vi "Read Lockin Digitizer Configuration.vi"(8 "error in (no error)":errorcluster, 11 "DAQmx RP I-V Driver in":refnum<class "RP I-V Driver.lvclass">) -> (0 "error out":errorcluster, 2 "Configuration":T1={"Post-trigger delay"=0.01, "Post-trigger duration"=0.1, "Rate"=1000000.0, "Ranges"=[10.0], "Re-name channels"=[], "Active channels"="0:1", "External\nclock"=FALSE, "Monitor time\nconstant"=1.0, "Sync"=FALSE, "Lock-in input channel phases"=[], "Output channels configuration"=[]} {"Output channels configuration"."Output amplitude" format="%#_6pV"; "Output channels configuration"."Frequency" format="%#_6pHz"; "Monitor time\nconstant" format="%#_6ps"; "Rate" format="%#_8pHz"; "Post-trigger duration" format="%#_6ps"; "Post-trigger delay" format="%#_6ps"; "Ranges" format="%#_6pV"}, 3 "DAQmx RP I-V Driver in":refnum<class "RP I-V Driver.lvclass">)   [LabVIEW 2024, in "RP I-V Driver.lvclass"]
uses:
  RP I-V Driver.lvclass
  Instruments/Pulse Driver/Lockin Digitizer Driver/Lockin Digitizer Configuration.ctl
  RP I-V Driver.lvclass/RP I-V Driver.ctl
  Instruments/Lockin Digitizer Driver/Output Channel Configuration.ctl
panel:
  # "Pulse config"
  # "Lock-in config"
  # "Output        Output          Input\nfrequency    amplitude    channels"
  # "#0\n\n#1\n\n#3"
  # "Monitor config"
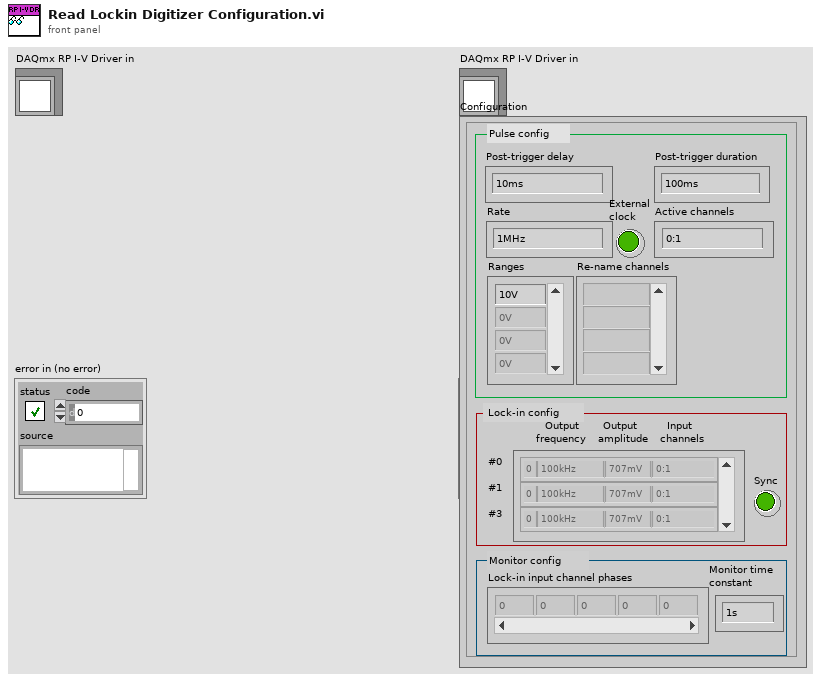
[diagram p1: front panel]
types:
  T1 = typedef "Lockin Digitizer Configuration.ctl" = cluster{"Post-trigger delay":dbl, "Post-trigger duration":dbl, "Rate":dbl, "Ranges":dbl[], "Re-name channels":string[], "Active channels":string, "External\nclock":bool, "Monitor time\nconstant":dbl, "Sync":bool, "Lock-in input channel phases":dbl[], "Output channels configuration":T2[]}
  T2 = typedef "Output Channel Configuration.ctl" = cluster{"Input channels":string, "Frequency":dbl, "Output amplitude":dbl, "Output channel number":i32}
  T3 = typedef "Pusle Driver Configuration.ctl" = cluster{"Post-trigger delay":dbl, "Post-trigger duration":dbl, "Rate":dbl, "Ranges":dbl[], "Re-name channels":string[], "Active channels":string, "External clock":bool}
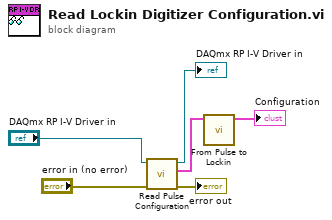
[diagram p0: block diagram]
diagram:
  n1 = call-dynamic "Read Pulse Configuration.vi"("error in (no error)"="error in (no error)", "RP I-V Driver in"="DAQmx RP I-V Driver in") -> ("error out"=→"error out":errorcluster, "Configuration"=w4:T3, "RP I-V Driver out"=→"DAQmx RP I-V Driver in":refnum<class "RP I-V Driver.lvclass">)  [unwired: 7 in]
  n2 = call "From Pulse to Lockin.vi"("Pulse Configuration in"=w4) -> ("Lockin Configuration out"=→"Configuration":T1)  [unwired: 10 in]
